vi "SQL_query.vi"(3 "error in (no error)":errorcluster, 4 "SQL query":string, 5 "联机模式":enum16{"单机", "联网"}(ring)=enum."联网") -> (0 "error out":errorcluster, 1 "data":string[][](array[string]), 2 "recordset reference out":T1)   [LabVIEW 2020]
uses:
  <vilib>/addons/database/Recordset.llb/Rec ObjectReference.ctl
  <vilib>/addons/database/Connection.llb/DB Tools Open Connec (String).vi
  <vilib>/addons/database/Connection.llb/Conn Execute.vi
  <vilib>/addons/database/Recordset.llb/Rec Fetch Recordset Data (R).vi
  <vilib>/addons/database/NI_Database_API.lvlib
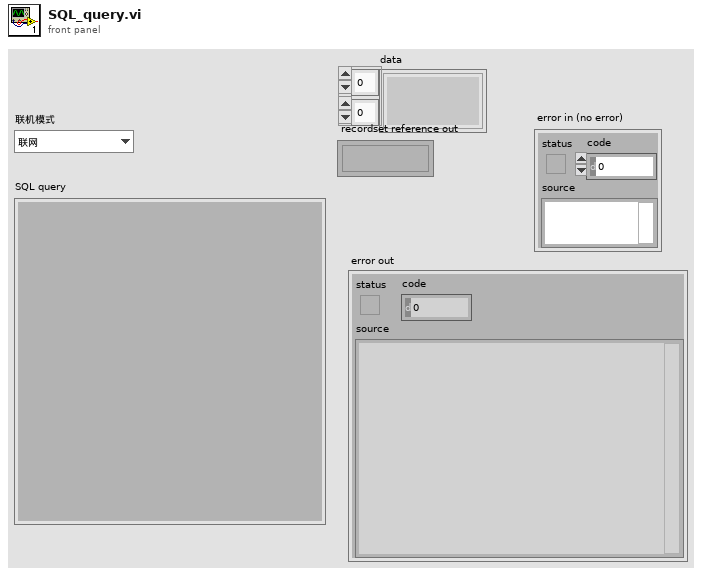
[diagram p1: front panel]
types:
  T1 = typedef "NI_Database_API.lvlib/Rec ObjectReference.ctl" = refnum<k1>
  T2 = typedef "NI_Database_API.lvlib/Conn ObjectReference.ctl" = refnum<k1>
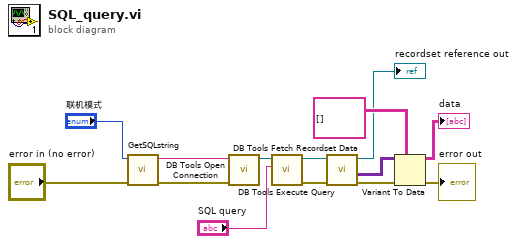
[diagram p0: block diagram]
diagram:
  n1 = call "GetSQLstring.vi"("错误输入"="error in (no error)", "联机模式"="联机模式") -> ("错误输出"=w2:errorcluster, "连接字符串"=w4:string)  [unwired: 8 in]
  n2 = call-poly <vilib>:"DB Tools Open Connection.vi"("error in (no error)"=w2, "connection information"=w4) -> ("connection reference"=w8:T2)  [unwired: 6 in, 1 out]
  n3 = call-poly <vilib>:"DB Tools Execute Query.vi"("SQL query"="SQL query", "connection reference"=w8) -> ("error out"=w14:errorcluster, "recordset reference"=w13:T1)  [unwired: 6 in]
  n4 = call-poly <vilib>:"DB Tools Fetch Recordset Data.vi"("error in (no error)"=w14, "recordset reference"=w13) -> ("error out"=w12:errorcluster, "recordset data"=w11:variant[][], "recordset reference out"=→"recordset reference out":T1)  [unwired: 3 in]
  n5 = Variant To Data(error in=w12, type=string[][] [], Variant=w11) -> (data=→"data":string[][], error out=→"error out":errorcluster)
